vi "PoseWithCurve_New.vi"(9 "POSE":T1={"TRANSLATION"={"X"=0.0, "Y"=0.0}, "ROTATION"={"VALUE"=0.0, "COS"=1.0, "SIN"=0.0}} {"ROTATION"."SIN" format="%13.4f"; "ROTATION"."COS" format="%13.4f"; "ROTATION"."VALUE" format="%13.4f"; "TRANSLATION"."Y" format="%14.3f"; "TRANSLATION"."X" format="%14.3f"}, 11 "CURVATURE":dbl) -> (3 "newPOSEwCURVATURE":T4={"CURVATURE"=0.0, "POSE"={"TRANSLATION"={"X"=0.0, "Y"=0.0}, "ROTATION"={"VALUE"=0.0, "COS"=1.0, "SIN"=0.0}}} {"POSE"."ROTATION"."SIN" format="%13.4f"; "POSE"."ROTATION"."COS" format="%13.4f"; "POSE"."ROTATION"."VALUE" format="%13.4f"; "POSE"."TRANSLATION"."Y" format="%14.3f"; "POSE"."TRANSLATION"."X" format="%14.3f"})   [LabVIEW 2019, in "Trajectory_Library.lvlib"]
doc: "Constructs a PoseWithCurvature.\n\nParameters:\n - pose - The pose. (Meters)\n - curvature - The curvature. (Radians/Meter)\n\nReturns:\n - NewPoseWCurvature - The PoseWCurvature data structure"
uses:
  Trajectory_Library.lvlib
  TypeDef/TRANSLATION2D.ctl
  TypeDef/ROTATION2D.ctl
  TypeDef/POSE2D.ctl
  TypeDef/POSEwCURVATURE.ctl
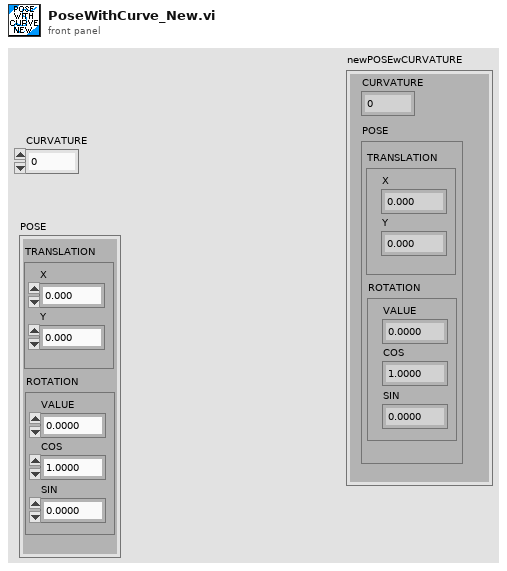
[diagram p1: front panel]
types:
  T1 = typedef "Trajectory_Library.lvlib/POSE2D.ctl" = cluster{"TRANSLATION":T2, "ROTATION":T3}
  T2 = typedef "Trajectory_Library.lvlib/TRANSLATION2D.ctl" = cluster{"X":dbl, "Y":dbl}
  T3 = typedef "Trajectory_Library.lvlib/ROTATION2D.ctl" = cluster{"VALUE":dbl, "COS":dbl, "SIN":dbl}
  T4 = typedef "Trajectory_Library.lvlib/POSEwCURVATURE.ctl" = cluster{"CURVATURE":dbl, "POSE":T1}
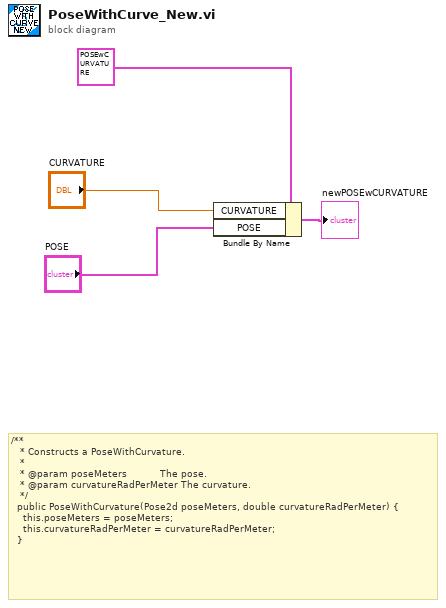
[diagram p0: block diagram]
diagram:
  # "/**\n   * Constructs a PoseWithCurvature.\n   *\n   * @param poseMeters           The pose.\n   * @param curvatureRadPerMeter The curvature.\n   */\n  public PoseWithCurvature(Pose2d poseMeters, double curvatureRadPerMeter) {\n    this.poseMeters = poseMeters;\n    this.curvatureRadPerMeter = curvatureRadPerMeter;\n  }"
  n1 = Bundle By Name(cluster=T4 {"CURVATURE"=0.0, "POSE"={"TRANSLATION"={"X"=0.0, "Y"=0.0}, "ROTATION"={"VALUE"=0.0, "COS"=1.0, "SIN"=0.0}}} ("POSEwCURVATURE"), "CURVATURE"="CURVATURE", "POSE"="POSE") -> (→"newPOSEwCURVATURE":T4)
